vi "RSZVB Set Chopped Pulse Profile Delay Increment.vi"(8 "error in (no error)":errorcluster {"code" format="%.0x"}, 9 "Delay Increment (0.0 s)":dbl format="%^.3e", 10 "Channel (1)":i32=1, 11 "VISA session":refnum<visa-resource-name>) -> (0 "error out":errorcluster {"code" format="%.0x"}, 3 "dup VISA session":refnum<visa-resource-name>)   [LabVIEW 2011]
doc: "This VI defines a delay increment for the sync signal in chopped pulse profile mode. The delay increment defines the distance between two measurement intervals (sweep points). For sweep point no. n, the total delay of thhe sync signal relative to the pulse generator signal is <Delay> + n * <Increment>.\n\nNote(s):\n\n(1) This VI is available only with option R&S ZVA-K27.\n\nRemote-control command(s):\n[SENSe<Ch>:]PULSe:GENerator<gen_no>:DINCrement"
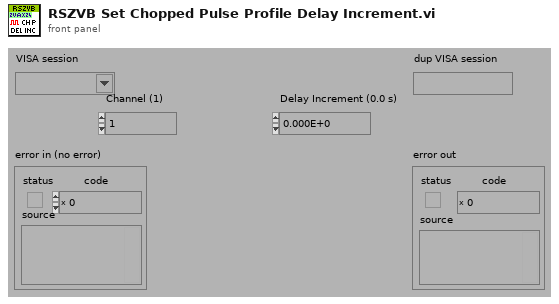
[diagram p1: front panel]
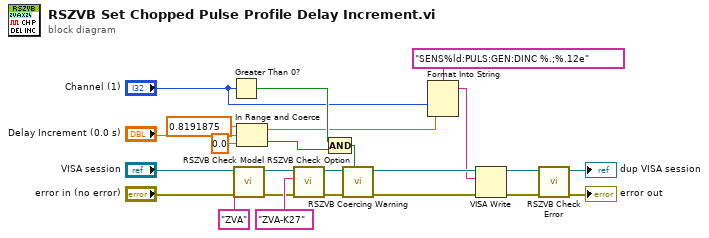
[diagram p0: block diagram]
diagram:
  n1 = Greater Than 0?(x="Channel (1)") -> (x > 0?=w8:bool)
  n2 = call "RSZVB Check Model.vi"("error in (no error)"="error in (no error)", "Model"="ZVA" ("Options"), "VISA session"="VISA session") -> ("error out"=w14:errorcluster, "dup VISA session"=w15:refnum<visa-resource-name>)  [unwired: 7 in]
  n3 = In Range and Coerce(upper limit=0.8191875, x="Delay Increment (0.0 s)", lower limit=0.0) -> (coerced(x)=w7:dbl, In Range?=w9:bool)
  n4 = call "RSZVB Check Option.vi"("error in (no error)"=w14, "Options"="ZVA-K27", "VISA session"=w15) -> ("error out"=w17:errorcluster, "dup VISA session"=w16:refnum<visa-resource-name>)  [unwired: 7 in]
  n5 = Compound Arithmetic op=AND(w8, w9) -> (w11:bool)
  n6 = call "RSZVB Coercing Warning.vi"("In Range?"=w11, "error in (no error)"=w17, "VISA session"=w16) -> ("error out"=w23:errorcluster, "dup VISA session"=w24:refnum<visa-resource-name>)  [unwired: 7 in]
  n7 = Format Into String(format string="SENS%ld:PULS:GEN:DINC %.;%.12e", "Channel (1)", w7) -> (resulting string=w20:string)  [unwired: 2 in, 1 out]
  n8 = VISA Write(VISA resource name=w24, write buffer=w20, error in (no error)=w23) -> (VISA resource name out=w21:refnum<visa-resource-name>, error out=w22:errorcluster)  [unwired: 1 out]
  n9 = call "RSZVB Check Error.vi"("error in (no error)"=w22, "VISA session"=w21) -> ("error out"=→"error out":errorcluster, "dup VISA session"=→"dup VISA session":refnum<visa-resource-name>)  [unwired: 8 in]
